vi "Blowfish F(X).vi"(1 "X":u32, 2 "S 4X256":u32[][](array[numeric])) -> (0 "F(X)":u32)   [LabVIEW 2020, in "Registration.lvclass"]
uses:
  Registration.lvclass
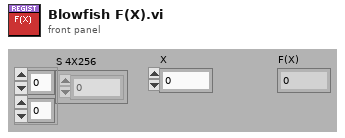
[diagram p1: front panel]
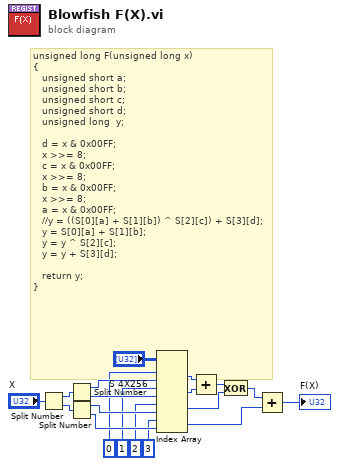
[diagram p0: block diagram]
diagram:
  # "unsigned long F(unsigned long x)\n{\n   unsigned short a;\n   unsigned short b;\n   unsigned short c;\n   unsigned short d;\n   unsigned long  y;\n\n   d = x & 0x00FF;\n   x >>= 8;\n   c = x & 0x00FF;\n   x >>= 8;\n   b = x & 0x00FF;\n   x >>= 8;\n   a = x & 0x00FF;\n   //y = ((S[0][a] + S[1][b]) ^ S[2][c]) + S[3][d];\n   y = S[0][a] + S[1][b];\n   y = y ^ S[2][c];\n   y = y + S[3][d];\n\n   return y;\n}"
  n1 = Split Number(x="X") -> (hi(x)=w2:u16, lo(x)=w3:u16)
  n2 = Split Number(x=w2) -> (hi(x)=w16:u8, lo(x)=w17:u8)
  n3 = Split Number(x=w3) -> (hi(x)=w18:u8, lo(x)=w19:u8)
  n4 = Index Array(array="S 4X256", index (row) #1=0 ("index (row)"), index (col) #1=w16, index (row) #2=1 ("index (row)"), index (col) #2=w17, index (row) #3=2 ("index (row)"), index (col) #3=w18, index (row) #4=3 ("index (row)"), index (col) #4=w19) -> (element #1=w9:u32, element #2=w10:u32, element #3=w12:u32, element #4=w14:u32)
  n5 = Add(x=w9, y=w10) -> (x+y=w11:u32)
  n6 = Exclusive Or(1:w12, 2:w11) -> (0:w13:u32)
  n7 = Add(x=w13, y=w14) -> (x+y=→"F(X)":u32)
